vi "Stop Module.vi"(6 "Timeout to Wait for Stop (s) (-1: no timeout)":dbl=-1.0, 8 "error in":errorcluster, 9 "Wait for Module to Stop? (F)":bool, 10 "Origin":string) -> (0 "error out":errorcluster)   [LabVIEW 2020, in "GUI.lvlib"]
doc: "Send the Stop request to the Module's Main.vi.\n\nIf <b>Wait for Module to Stop?</b> is TRUE, this VI will wait until the module main VI stops, and will timeout at the <b>Timeout to Wait for Stop</b> value. This value defaults to \"-1\", which means the VI will not timeout, and will always wait until the module main VI stops before completing execution.\n\nNote: The <b>Timeout to Wait for Stop</b> value is ignored if 'Wait for Module to Stop?' is set to FALSE.\n_____\nBased on DQMH Project Template 6.1.0.94."
uses:
  GUI.lvlib
  Stop Argument--cluster.ctl
  <vilib>/event_ctls.llb/usereventprio.ctl
panel:
  # "Note: The 'Timeout to Wait for Stop' value is ignored if 'Wait for Module to Stop?' is set to FALSE."
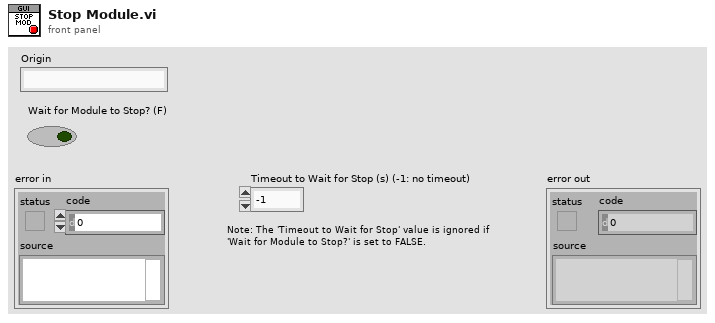
[diagram p1: front panel]
types:
  T1 = typedef "GUI.lvlib/Stop Argument--cluster.ctl" = cluster{"Origin":string, "Exit via Stop Module Req?":bool, "Wait for Module to stop?":bool}
  T2 = typedef "usereventprio.ctl" = enum32{"high priority", "normal priority"}
  T3 = typedef "GUI.lvlib/Request Events--cluster.ctl" = cluster{"Stop Module":refnum<user-event>, "Show Panel":refnum<user-event>, "Hide Panel":refnum<user-event>, "Get Module Execution Status":refnum<user-event>, "Show Diagram":refnum<user-event>}
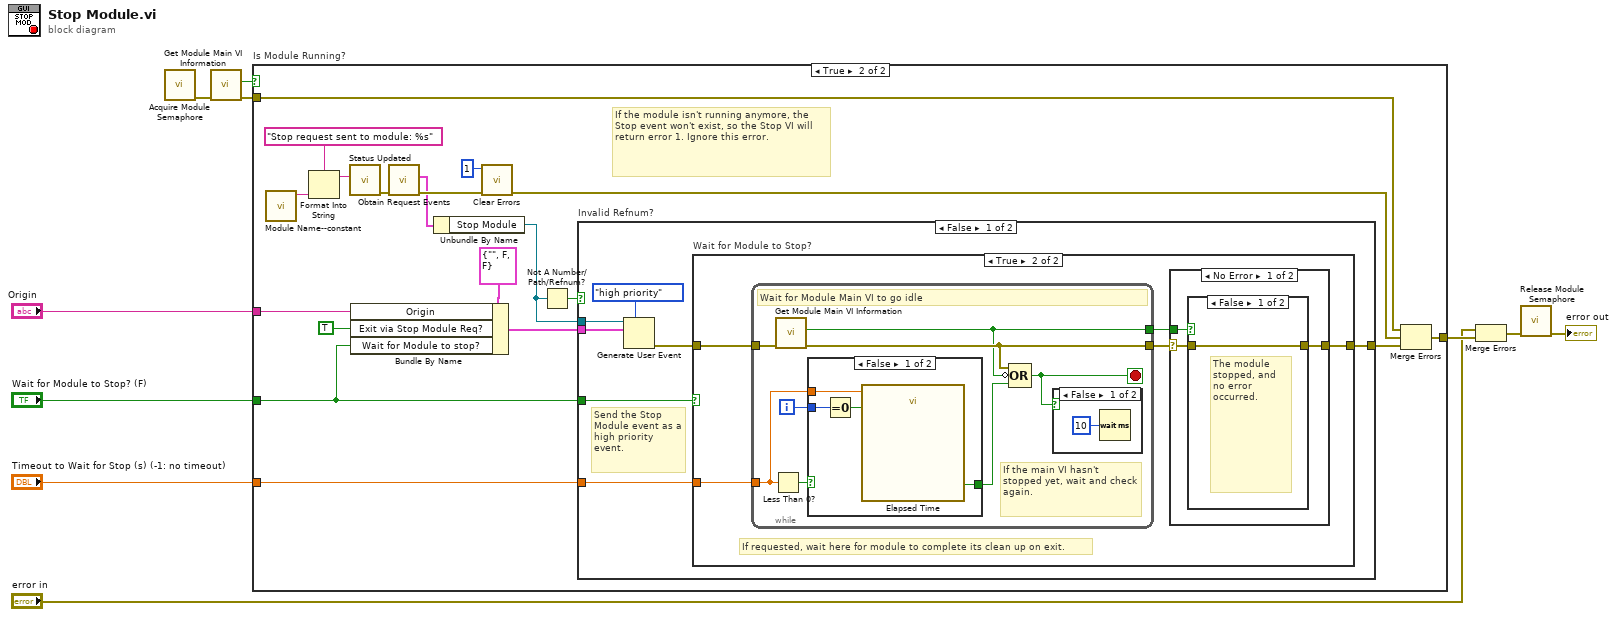
[diagram p0: block diagram]
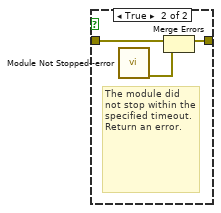
[diagram p4: hidden frame]
diagram:
  n1 = call "Acquire Module Semaphore.vi"() -> ("error out"=w4:errorcluster)  [unwired: 11 in]
  n2 = call "Get Module Main VI Information.vi"("error in"=w4) -> ("error out"=w7:errorcluster, "Is Module Running?"=w6:bool)  [unwired: 7 in, 2 out]
  n3 = case "Is Module Running?" shown="True" w6 {
    tunnel: [w11 w29] -> w10
    tunnel: "Origin" -> [_ w28]
    tunnel: w7 -> [w11 w17]
    tunnel: "Wait for Module to Stop? (F)" -> [_ w13]
    tunnel: "Timeout to Wait for Stop (s) (-1: no timeout)" -> [_ w12]
    frame False {
      # "The module is not running, there is no need to run the Stop Module code."
    }
    frame True {
      # "If the module isn't running anymore, the Stop event won't exist, so the Stop VI will return error 1. Ignore this error."
      n4 = call "Module Name--constant.vi"() -> ("Module Name"=w24:string)  [unwired: 11 in]
      n5 = Format Into String(format string="Stop request sent to module: %s", w24) -> (resulting string=w25:string)  [unwired: 2 in, 1 out]
      n6 = call "Status Updated.vi"("Status"=w25) -> ("error out"=w16:errorcluster)  [unwired: 10 in]
      n7 = Bundle By Name(cluster=T1 {"Origin"="", "Exit via Stop Module Req?"=FALSE, "Wait for Module to stop?"=FALSE} ("event data"), "Origin"=w28, "Exit via Stop Module Req?"=TRUE, "Wait for Module to stop?"=w13) -> (w20:T1)
      n8 = call "Obtain Request Events.vi"("error in (no error)"=w16) -> ("error out"=w30:errorcluster, "GUI Request Events"=w27:T3)  [unwired: 9 in]
      n9 = Unbundle By Name(w27) -> ("Stop Module"=w21:refnum<user-event>)
      n10 = call <vilib>:"Clear Errors.vi"("error in (no error)"=w30, "specific error code to clear (0: all)"=1) -> ("error out"=w15:errorcluster)  [unwired: 4 in, 1 out]
      n11 = Not A Number/Path/Refnum?(number/path/refnum=w21) -> (NaN/Path/Refnum?=w22:bool)
      n12 = case "Invalid Refnum?" shown="False" w22 {
        tunnel: [w32 _] -> w19
        tunnel: w21 -> [w37 _]
        tunnel: w20 -> [w35 _]
        tunnel: w13 -> [w33 _]
        tunnel: w12 -> [w31 _]
        frame False {
          # "Send the Stop Module event as a high priority event."
          n13 = Generate User Event(priority (normal)=usereventprio."high priority", user event=w37, event data cluster=w35) -> (error out=w34:errorcluster)  [unwired: 1 in, 1 out]
          n14 = case "Wait for Module to Stop?" shown="True" w33 {
            tunnel: w34 -> [w38 w42]
            tunnel: [w38 w40] -> w32
            tunnel: w31 -> [_ w43]
            frame False {
            }
            frame True {
              # "If requested, wait here for module to complete its clean up on exit."
              n15 = while {
                tunnel: w43 -> [w54]
                tunnel: w42 -> [w58]
                tunnel: [w57] -> w41
                tunnel: [w56] -> w39
                i -> [w59]
                stop <- w52 stop-if-true
                # "If the main VI hasn't stopped yet, wait and check again."
                # "Wait for Module Main VI to go idle"
                n16 = Less Than 0?(x=w54) -> (x < 0?=w53:bool)
                n17 = call "Get Module Main VI Information.vi"("error in"=w58) -> ("error out"=w57:errorcluster, "Is Module Running?"=w56:bool)  [unwired: 7 in, 2 out]
                n18 = case shown="False" w53 {
                  tunnel: w54 -> [w61 _]
                  tunnel: w59 -> [w63 _]
                  tunnel: [w62 _] -> w55
                  frame False {
                    n19 = Equal To 0?(x=w63) -> (x = 0?=w64:bool)
                    n20 = call "Elapsed Time"("Time Target (s)"=w61, "Reset"=w64) -> ("Time has Elapsed"=w62:bool)  [unwired: 10 in, 7 out]
                  }
                  frame True {
                    # "User specified a timeout of -1, so don't keep track of the elapsed time since this loop started."
                  }
                }
                n21 = Compound Arithmetic op=OR(w57, invert w56, w55) -> (w52:bool)
                n22 = case shown="False" w52 {
                  frame False {
                    n23 = Wait (ms)(milliseconds to wait=u32 10) -> ()  [unwired: 1 out]
                  }
                  frame True {
                  }
                }
              }
              n24 = case shown="No Error" w41 {
                selector: w41 -> [w45 w51]
                tunnel: [w44 w51] -> w40
                tunnel: w39 -> [w46 _]
                frame No Error {
                  n25 = case shown="False" w46 {
                    tunnel: w45 -> [w47 w50]
                    tunnel: [w47 w49] -> w44
                    frame False {
                      # "The module stopped, and no error occurred."
                    }
                    frame True {
                      # "The module did not stop within the specified timeout. Return an error."
                      n26 = call "Module Not Stopped--error.vi"() -> ("error out"=w48:errorcluster)  [unwired: 11 in]
                      n27 = Merge Errors(w50, w48) -> (w49:errorcluster)
                    }
                  }
                }
                frame Error {
                  # "An error occurred while waiting for the module to stop. Return that error."
                }
              }
            }
          }
        }
        frame True {
          # "Module is exiting. No need to send the standard \"not running\" error that is sent in other request VIs."
        }
      }
      n28 = Merge Errors(w17, w15, w19) -> (w29:errorcluster)
    }
  }
  n29 = Merge Errors("error in", w10) -> (w2:errorcluster)
  n30 = call "Release Module Semaphore.vi"("error in"=w2) -> ("error out"=→"error out":errorcluster)  [unwired: 10 in]
